vi "rqp_Write CMD.vi"(4 "Show in Debugger?":bool=TRUE, 6 "Message Priority":T1=enum."Normal", 7 "Caller in":refnum<class "Worker.lvclass">, 8 "error in":errorcluster, 10 "Data in":T2 {"CMD"."Mix_CMD" items=["Мешалка движение вперёд"=1, "Мешалка движение назад"=2, "Мешалка стоп"=9]; "CMD"."Termex_CMD" items=["Термостат старт"=1, "Термостат стоп"=9]; "CMD"."Rotate_CMD" items=["Качалка Дом"=1, "Качалка Режим Авто - Старт"=2, "Качалка Режим Ручной - Старт"=3, "Качалка Стоп"=9]}, 11 "gui in":refnum<class "gui.lvclass">) -> (0 "error out":errorcluster, 3 "dup gui out":refnum<class "gui.lvclass">, 5 "dup Caller out":refnum<class "Worker.lvclass">)   [LabVIEW 2023, in "GUI.lvlib" / "gui.lvclass"]
doc: "This VI sends a <b>Public API Request</b> message to an MHL case of the Worker that owns this VI.\n---\nWorkers Public API Request Case"
uses:
  gui.lvclass
  C:/Program Files/National Instruments/LabVIEW 2023/vi.lib/addons/_Workers/Library/Classes/Worker/Worker.lvclass
  <vilib>/addons/_Workers/Library/Classes/Worker/Worker.lvclass
  rqp_Write CMD.ctl
  Modbus PLC/Modbus PLC/Commands.ctl
  <vilib>/addons/_Workers/Library/Classes/Message/Priority.ctl
  <vilib>/addons/_Workers/Library/Case Label.ctl
  <vilib>/addons/_Workers/Library/Classes/Message Queue/Message Queue.lvclass
  <vilib>/addons/_Workers/Library/Workers.lvlib
  <vilib>/addons/_Workers/Library/Classes/Message/Message.lvclass
  Modbus PLC/Modbus PLC/Modbus PLC.lvclass
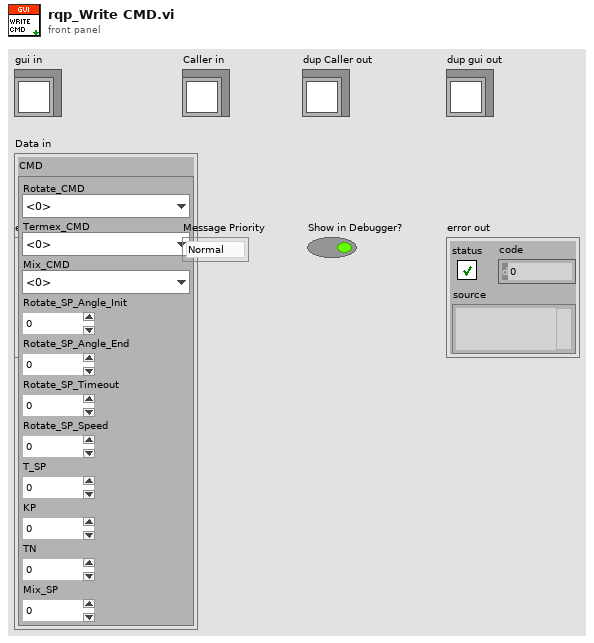
[diagram p1: front panel]
types:
  T1 = typedef "Workers.lvlib/Message.lvclass/Priority.ctl" = enum16{"Low", "Normal", "High"}
  T2 = typedef "GUI.lvlib/gui.lvclass/rqp_Write CMD.ctl" = cluster{"CMD":T3}
  T3 = typedef "Modbus PLC.lvlib/Modbus PLC.lvclass/Commands.ctl" = cluster{"Rotate_CMD":u16, "Termex_CMD":u16, "Mix_CMD":u16, "Rotate_SP_Angle_Init":u16, "Rotate_SP_Angle_End":u16, "Rotate_SP_Timeout":u16, "Rotate_SP_Speed":u16, "T_SP":sgl, "KP":sgl, "TN":sgl, "Mix_SP":u16}
  T4 = typedef "Workers.lvlib/Case Label.ctl" = string
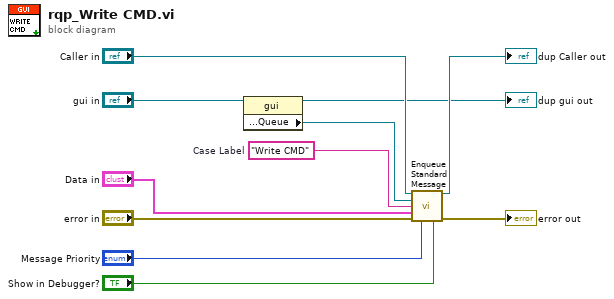
[diagram p0: block diagram]
diagram:
  w1 = T4 "Write CMD"  # Case Label
  n1 = property class="gui"(reference="gui in") -> (reference out=→"dup gui out":refnum<class "gui.lvclass">, "Accessors:Read:Public API:Queue"=w2:refnum<class "Message Queue.lvclass">)  [unwired: 1 in, 1 out]
  n2 = call-dynamic "Enqueue Standard Message.vi"("Worker"="Caller in", "Message Queue"=w2, "Case Label"=w1, "Data"="Data in", "error in (no error)"="error in", "Priority (Normal)"="Message Priority", "Send Message to Debugger? (T)"="Show in Debugger?") -> ("dup Worker out"=→"dup Caller out":refnum<class "Worker.lvclass">, "error out"=→"error out":errorcluster)  [unwired: 7 in]
